vi "f24.vi"() -> ()   [LabVIEW 2014]
panel:
  in  "f24":dbl
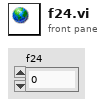
[diagram p1: front panel]
diagram:
